vi "Battery Level Test.vi"   [LabVIEW 2012]
uses:
  <vilib>/Rock Robotics/SystemInterfaces/Typedef/FPGA_TypedefAnalogModule.ctl
  <vilib>/Rock Robotics/SystemInterfaces/AI/FPGA_AIChannel.ctl
  <vilib>/Rock Robotics/SystemInterfaces/Typedef/FPGA_TypedefDigitalModule.ctl
  Robot Global Data.vi
types:
  T1 = typedef "FPGA_AIChannel.ctl" = enum8{"AI 1", "AI 2", "AI 3", "AI 4", "AI 5", "AI 6", "AI 7", "AI 8", "Invalid"}
  T2 = typedef "FPGA_TypedefAnalogModule.ctl" = enum16{"Analog Module 1", "Analog Module 2"}
  T3 = typedef "WPI_AnalogChannelDevRef.ctl" = cluster{"DevStatus":errorcluster, "Analog Module":T2, "Analog Channel":T1}
  T4 = typedef "FPGA_TypedefDigitalModule.ctl" = enum16{"Digital Module 1", "Digital Module 2"}
  T5 = enum16{"FOUR_ZONES", "ONE_ZONE_TWO_LINES", "TWO_ZONES_ONE_LINE"}
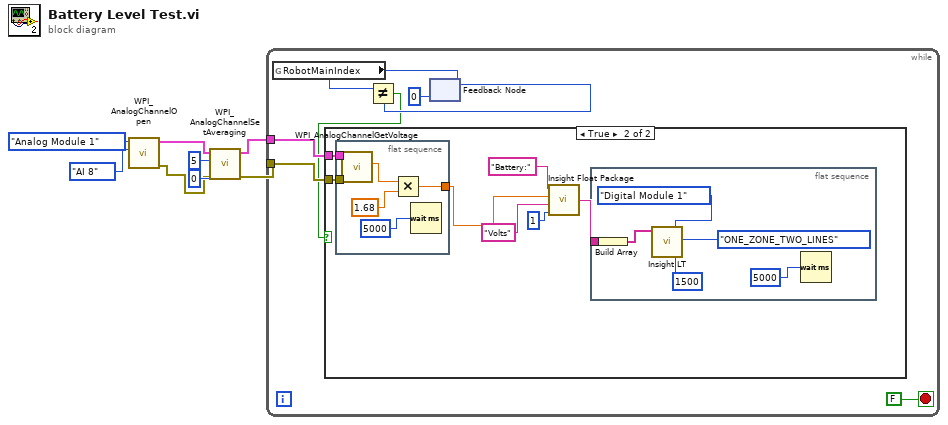
[diagram p0: block diagram]
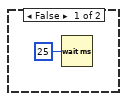
[diagram p2: hidden frame]
diagram:
  n1 = call <vilib>:"WPI_AnalogChannelOpen.vi"("Analog Channel"=FPGA_AIChannel."AI 8", "Analog Module (Module 1)"=FPGA_TypedefAnalogModule."Analog Module 1") -> ("error out"=w4:errorcluster, "AIDeviceRef"=w3:T3)  [unwired: 8 in]
  n2 = call <vilib>:"WPI_AnalogChannelSetAveraging.vi"("error in (no error)"=w4, "OversampleBits"=u8 0, "AverageBits"=u8 5, "AIDeviceRef"=w3) -> ("error out"=w1:errorcluster, "AIDeviceRef"=w2:T3)  [unwired: 6 in]
  n3 = while {
    tunnel: w1 -> [w14]
    tunnel: w2 -> [w13]
    stop <- FALSE stop-if-true
    n4 = global read "Robot Global Data.vi" "RobotMainIndex"() -> (w11:i32)
    n5 = feedback #1(0 ("TeleopIndex")) -> (w12:i32)
    n6 = Not Equal?(x=w11, y=w12) -> (x != y?=w9:bool)
    n7 = case shown="True" w9 {
      tunnel: w14 -> [_ w22]
      tunnel: w13 -> [_ w21]
      frame False {
        n8 = Wait (ms)(milliseconds to wait=u32 25) -> ()  [unwired: 1 out]
      }
      frame True {
        n9 = flat-sequence {
          tunnel: w22 -> [w33]
          tunnel: w21 -> [w32]
          tunnel: [w31] -> w20
          frame #0 {
            n10 = call <vilib>:"WPI_AnalogChannelGetVoltage.vi"("error in (no error)"=w33, "AIDeviceRef"=w32) -> ("Voltage"=w35:dbl)  [unwired: 7 in, 2 out]
            n11 = Multiply(x=w35, y=1.68) -> (x*y=w31:dbl)
            n12 = Wait (ms)(milliseconds to wait=u32 5000) -> ()  [unwired: 1 out]
          }
        }
        n13 = call "Insight Float Package.vi"("Decimal Places"=1, "Footer"="Volts", "Float"=w20, "Header"="Battery:") -> ("resulting string"=w23:string)
        n14 = flat-sequence {
          tunnel: w23 -> [w29]
          frame #0 {
            n15 = Build Array(w29) -> (w28:string[])
            n16 = call "Insight LT.vi"("Scroll Timing"=1500, "ZONE \nCONFIGURATION"=T5."ONE_ZONE_TWO_LINES" ("ZONE \nCONFIGURATION"), "Digital Module"=FPGA_TypedefDigitalModule."Digital Module 1", "Zone 1 Data"=w28) -> ()  [unwired: 3 in]
            n17 = Wait (ms)(milliseconds to wait=u32 5000) -> ()  [unwired: 1 out]
          }
        }
      }
    }
    n18 = feedback-in #1(w11) -> ()
  }
